vi "Connect.vi"(8 "error in (no error)":errorcluster, 9 "timeout":i32=-1, 11 "Error Stream in":refnum<class "Error Stream.lvclass">) -> (0 "error out":errorcluster, 3 "Error Stream out":refnum<class "Error Stream.lvclass">)   [LabVIEW 2020, in "Error Stream.lvclass"]
doc: "Override this method to specify the action the local copy of this object will perform to connect to its remote counterpart."
uses:
  Error Stream.lvclass
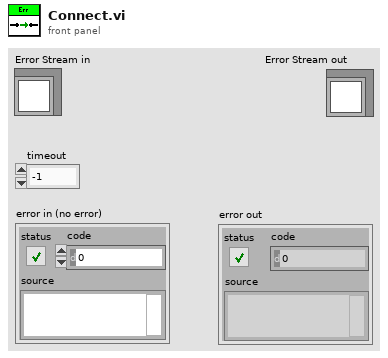
[diagram p1: front panel]
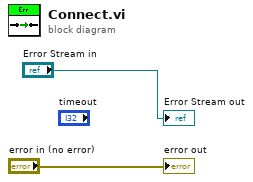
[diagram p0: block diagram]
diagram:
  "Error Stream out" <- "Error Stream in"
  "error out" <- "error in (no error)"
